vi "Revision Query Core.vi"(8 "error in (no error)":errorcluster, 11 "BNT_DAQmx-MCSV in":refnum<class "BNT_DAQmx-MCSV.lvclass">) -> (0 "error out":errorcluster, 1 "Firmware Revision":string, 2 "Driver Revision":string, 3 "BNT_DAQmx-MCSV out":refnum<class "BNT_DAQmx-MCSV.lvclass">)   [LabVIEW 2017, in "BNT_DAQmx.lvlib" / "BNT_DAQmx-MCSV.lvclass"]
uses:
  BNT_DAQmx-MCSV.lvclass
  BNT_DAQmx-MCSV.lvclass/BNT_DAQmx-MCSV.ctl
  CSPP_Core/Actors/CS++DeviceActor/CS++DeviceActor.lvclass
  <resource>/objmgr/daqmx.rc
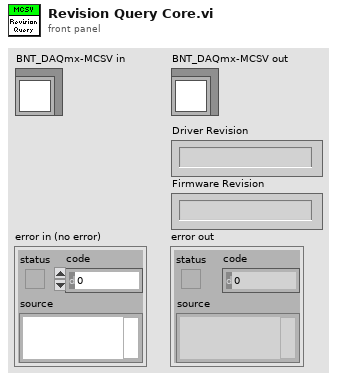
[diagram p1: front panel]
types:
  T1 = cluster{"Major":u16, "Minor":u16, "Fix":u16, "Build":u16}
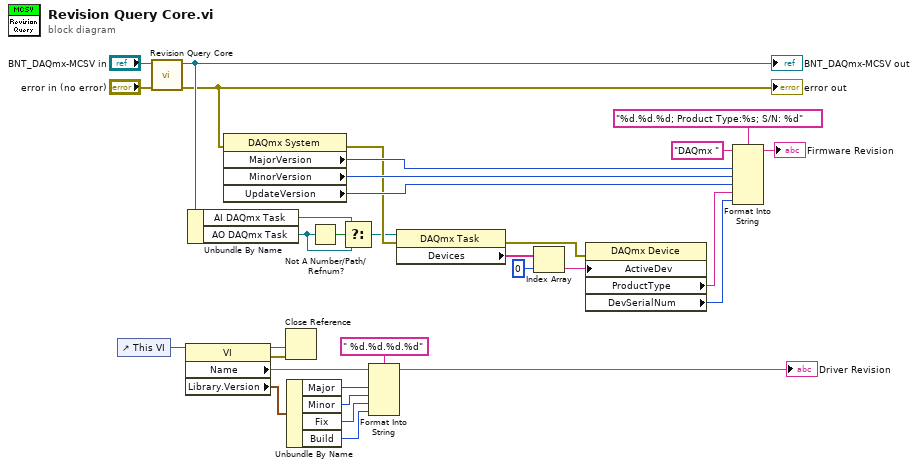
[diagram p0: block diagram]
diagram:
  n1 = control-ref of="This VI"() -> (w15:refnum<vi>)
  n2 = call-parent "Revision Query Core.vi"("error in (no error)"="error in (no error)", "CS++DeviceActor in"="BNT_DAQmx-MCSV in") -> ("error out"=w21:errorcluster, "CS++DeviceActor out"=w30:refnum<class "BNT_DAQmx-MCSV.lvclass">)  [unwired: 6 in, 2 out]
  "error out" <- w21
  "BNT_DAQmx-MCSV out" <- w30
  n3 = property class="VI"(reference=w15) -> (reference out=w13:refnum<vi>, error out=w14:errorcluster, "Name"=w10:string, "Library.Version"=w12:T1)  [unwired: 1 in]
  n4 = Unbundle By Name(w30) -> ("AI DAQmx Task"=w2:refnum<k21>, "AO DAQmx Task"=w3:refnum<k21>)
  n5 = property class="DAQmx System"(error in=w21) -> (error out=w20:errorcluster, "MajorVersion"=w26:u32, "MinorVersion"=w25:u32, "UpdateVersion"=w24:u32)  [unwired: 1 in, 1 out]
  n6 = Close Reference(reference=w13, error in (no error)=w14) -> ()  [unwired: 1 out]
  n7 = Unbundle By Name(w12) -> ("Major"=w9:u16, "Minor"=w8:u16, "Fix"=w7:u16, "Build"=w6:u16)
  n8 = Not A Number/Path/Refnum?(number/path/refnum=w3) -> (NaN/Path/Refnum?=w4:bool)
  n9 = Select(t=w2, s=w4, f=w3) -> (s? t:f=w1:refnum<k21>)
  n10 = Format Into String(format string=" %d.%d.%d.%d" ("Driver Revision"), initial string=w10, w9, w8, w7, w6) -> (resulting string=→"Driver Revision":string)  [unwired: 1 in, 1 out]
  n11 = property class="DAQmx Task"(reference=w1, error in=w20) -> (error out=w19:errorcluster, "Devices"=w29:tag[])  [unwired: 1 out]
  n12 = Index Array(array=w29, index=0) -> (element=w27:tag)
  n13 = property class="DAQmx Device"(error in=w19, "ActiveDev"=w27) -> ("ProductType"=w18:string, "DevSerialNum"=w17:u32)  [unwired: 1 in, 2 out]
  n14 = Format Into String(format string="%d.%d.%d; Product Type:%s; S/N: %d", initial string="DAQmx ", w26, w25, w24, w18, w17) -> (resulting string=→"Firmware Revision":string)  [unwired: 1 in, 1 out]
